vi "continuous_AI.vi"() -> ()   [LabVIEW 2017]
uses:
  <vilib>/Utility/error.llb/DialogType.ctl
  <vilib>/DAQmx/read.llb/DAQmx Read (Analog 1D DBL 1Chan NSamp).vi
  <vilib>/DAQmx/create/channels.llb/DAQmx Create Channel (AI-Voltage-Basic).vi
  <vilib>/DAQmx/configure/timing.llb/DAQmx Timing (Sample Clock).vi
  <vilib>/DAQmx/configure/trigger.llb/DAQmx Start Trigger (None).vi
  <vilib>/DAQmx/miscellaneous.llb/DAQmx Fill In Error Info.vi
  <resource>/objmgr/daqmx.rc
panel:
  out "ms passed":u32
  in  "ms to wait":u32=100
  out "error out":errorcluster
  in  "stop":bool
  out "SpectrumGraph":cluster{i32[], dbl[]}(graph)
  out "AI.Max 2":dbl
  out "AI.Min 2":dbl
  in  "AI.Max":dbl=1.0
  in  "samples per channel":i32=500000
  in  "rate":dbl=100000.0 format="%0.0f"
  in  "DAQ channel (in)":tag="DAQ6363/ai2"
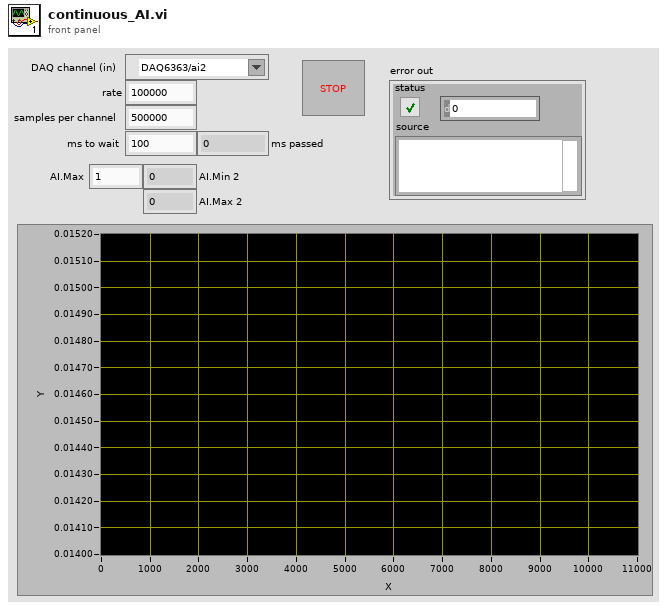
[diagram p1: front panel]
types:
  T1 = typedef "DialogType.ctl" = u16
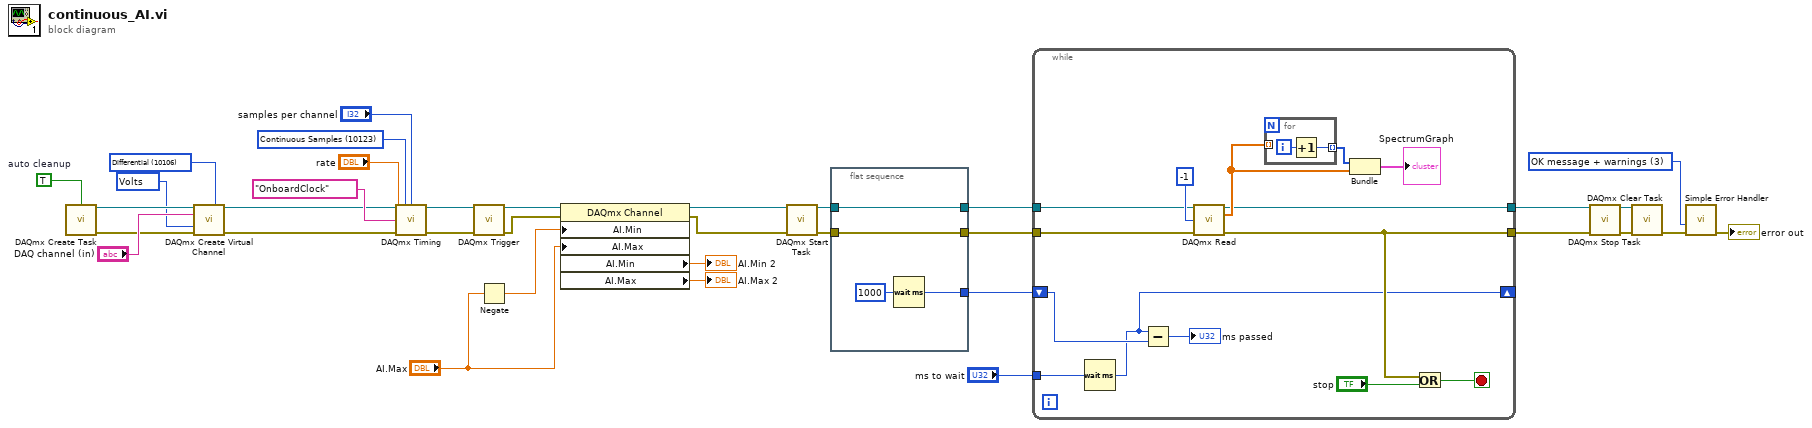
[diagram p0: block diagram]
diagram:
  w12 = T1 3 items=["no dialog", "OK message", "continue or stop message", "OK message + warnings", "continue/stop + warnings"] ("type of dialog (OK msg:1)")
  w32 = TRUE  # auto cleanup
  w34 = 10123 items=["Finite Samples"=10178, "Continuous Samples"=10123, "Hardware Timed Single Point"=12522] ("sample mode")
  w25 = 10106 items=["Default"=-1, "RSE"=10083, "NRSE"=10078, "Differential"=10106, "Pseudodifferential"=12529] ("input terminal configuration")
  w24 = 10348 items=["Volts"=10348, "From Custom Scale"=10065] ("units")
  n1 = call <vilib>:"DAQmx Create Task.vi"("auto cleanup"=w32) -> ("task out"=w31:refnum<k21>, "error out"=w30:errorcluster)  [unwired: 13 in]
  n2 = call-poly <vilib>:"DAQmx Create Virtual Channel.vi"("task in"=w31, "input terminal configuration"=w25, "physical channels"="DAQ channel (in)", "units"=w24, "error in"=w30) -> ("task out"=w23:refnum<k21>, "error out"=w22:errorcluster)  [unwired: 9 in]
  n3 = call-poly <vilib>:"DAQmx Timing.vi"("task/channels in"=w23, "sample mode"=w34, "samples per channel"="samples per channel", "rate"="rate", "source"=tag "OnboardClock", "error in"=w22) -> ("task out"=w29:refnum<k21>, "error out"=w28:errorcluster)  [unwired: 8 in]
  n4 = call-poly <vilib>:"DAQmx Trigger.vi"("task/channels in"=w29, "error in"=w28) -> ("task out"=w21:refnum<k21>, "error out"=w20:errorcluster)  [unwired: 12 in]
  n5 = Negate(x="AI.Max") -> (-x=w3:dbl)
  n6 = property class="DAQmx Channel"(reference=w21, error in=w20, "AI.Min"=w3, "AI.Max"="AI.Max") -> (reference out=w15:refnum<k21>, error out=w14:errorcluster, "AI.Min"=→"AI.Min 2":dbl, "AI.Max"=→"AI.Max 2":dbl)
  n7 = call <vilib>:"DAQmx Start Task.vi"("task/channels in"=w15, "error in"=w14) -> ("task out"=w17:refnum<k21>, "error out"=w16:errorcluster)  [unwired: 12 in]
  n8 = flat-sequence {
    tunnel: w16 -> [w39]
    tunnel: [w39] -> w7
    tunnel: w17 -> [w38]
    tunnel: [w38] -> w8
    tunnel: [w36] -> w2
    frame #0 {
      n9 = Wait (ms)(milliseconds to wait=u32 1000) -> (millisecond timer value=w36:u32)
    }
  }
  n10 = while {
    tunnel: w8 -> [w48]
    tunnel: w7 -> [w49]
    tunnel: [w46] -> w6
    tunnel: [w44] -> w5
    shift-right: [w40] -> _
    shift-left: w2 -> [w42]
    tunnel: "ms to wait" -> [w43]
    stop <- w45 stop-if-true
    n11 = Wait (ms)(milliseconds to wait=w43) -> (millisecond timer value=w40:u32)
    n12 = Subtract(x=w40, y=w42) -> (x-y=→"ms passed":u32)
    n13 = call-poly <vilib>:"DAQmx Read.vi"("task/channels in"=w48, "number of samples per channel"=-1, "error in"=w49) -> ("task out"=w44:refnum<k21>, "data"=w51:dbl[], "error out"=w46:errorcluster)  [unwired: 10 in]
    n14 = for {
      tunnel: [w54] -> w52 mode=indexing
      tunnel: w51 -> [_] mode=indexing
      i -> [w55]
      n15 = Increment(x=w55) -> (x+1=w54:i32)
    }
    n16 = Bundle(w52, "data"=w51) -> (→"SpectrumGraph":cluster{i32[], "data":dbl[]})  [unwired: 1 in]
    n17 = Or(x=w46, y="stop") -> (x .or. y?=w45:bool)
  }
  n18 = call <vilib>:"DAQmx Stop Task.vi"("task/channels in"=w5, "error in"=w6) -> ("task out"=w10:refnum<k21>, "error out"=w11:errorcluster)  [unwired: 12 in]
  n19 = call <vilib>:"DAQmx Clear Task.vi"("task in"=w10, "error in"=w11) -> ("error out"=w9:errorcluster)  [unwired: 13 in]
  n20 = call <vilib>:"Simple Error Handler.vi"("type of dialog (OK msg:1)"=w12, "error in (no error)"=w9) -> ("error out"=→"error out":errorcluster)  [unwired: 3 in, 4 out]
